vi "pid resistor simulation.vi"() -> ()   [LabVIEW 2020]
uses:
  <vilib>/addons/control/pid/pid.llb/PID (DBL).vi
  <vilib>/addons/control/pid/NI_PID_pid.lvlib
panel:
  in  "R":dbl
  out "XY Graph":cluster{dbl[], dbl[]}(graph)
  in  "PID gains":T1={"proportional gain (Kc)"=1.0, "integral time (Ti, min)"=0.01, "derivative time (Td, min)"=0.0} {"derivative time (Td, min)" format="%.3f"; "integral time (Ti, min)" format="%.3f"; "proportional gain (Kc)" format="%.3f"}
  out "output":dbl format="%.2f"
  in  "setpoint":dbl format="%.2f"
  in  "stop":bool
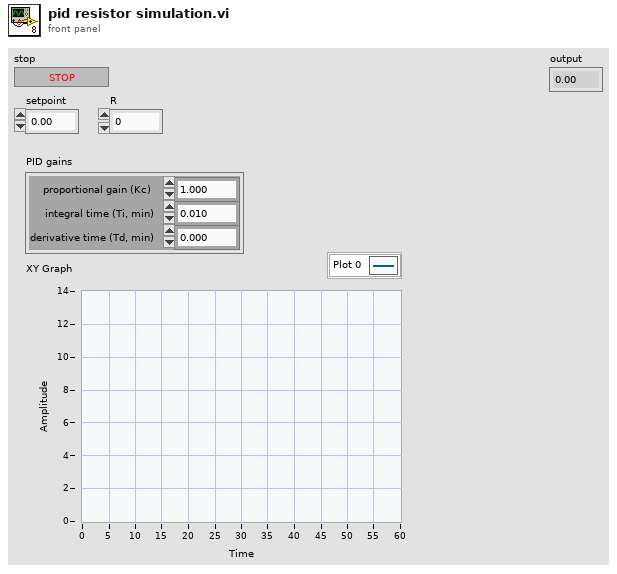
[diagram p1: front panel]
types:
  T1 = cluster{"proportional gain (Kc)":dbl, "integral time (Ti, min)":dbl, "derivative time (Td, min)":dbl}
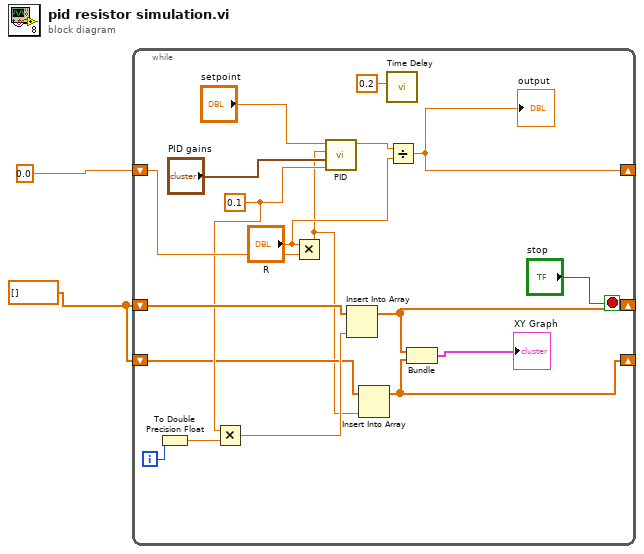
[diagram p0: block diagram]
diagram:
  w1 = dbl[] []
  n1 = while {
    shift-right: [w14] -> _
    shift-left: 0.0 ("output") -> [w17]
    shift-right: [w6] -> _
    shift-left: w1 -> [w13]
    shift-right: [w5] -> _
    shift-left: w1 -> [w8]
    i -> [w12]
    stop <- "stop" stop-if-true
    w10 = 0.1 ("dt (s)")
    n2 = To Double Precision Float(number=w12) -> (double precision float=w11:dbl)
    n3 = Multiply(x=w10, y=w11) -> (x*y=w9:dbl)
    n4 = Multiply(x="R", y=w17) -> (x*y=w7:dbl)
    n5 = call-poly <vilib>:"PID.vi"("dt (s)"=w10, "PID gains"="PID gains", "process variable"=w7, "setpoint"="setpoint") -> ("output"=w16:dbl)  [unwired: 6 in, 1 out]
    n6 = Insert Into Array(array=w13, new element=w9) -> (w6:dbl[])  [unwired: 1 in]
    n7 = Insert Into Array(array=w8, new element=w7) -> (w5:dbl[])  [unwired: 1 in]
    n8 = call "Time Delay"("Delay Time (s)"=0.2) -> ()  [unwired: 10 in, 1 out]
    n9 = Divide(x=w16, y="R") -> (x/y=w14:dbl)
    "output" <- w14
    n10 = Bundle(w6, w5) -> (→"XY Graph":cluster{dbl[], dbl[]})  [unwired: 1 in]
  }
